vi "Picture_View_ROI.vi"(8 "Input Cluster":T6, 10 "ROI":bool, 11 "Cluster 2":T7) -> (0 "ROI-Picture":i32[][](array[numeric]), 3 "Out of range":bool[](array[boolean]))   [LabVIEW 2009]
uses:
  atmcd32d.llb/AcquisitionMode_mode typedef.ctl
  atmcd32d.llb/ReadMode_mode typedef.ctl
  atmcd32d.llb/TriggerMode_mode typedef.ctl
  atmcd32d.llb/Shutter_type typedef.ctl
  atmcd32d.llb/Shutter_mode typedef.ctl
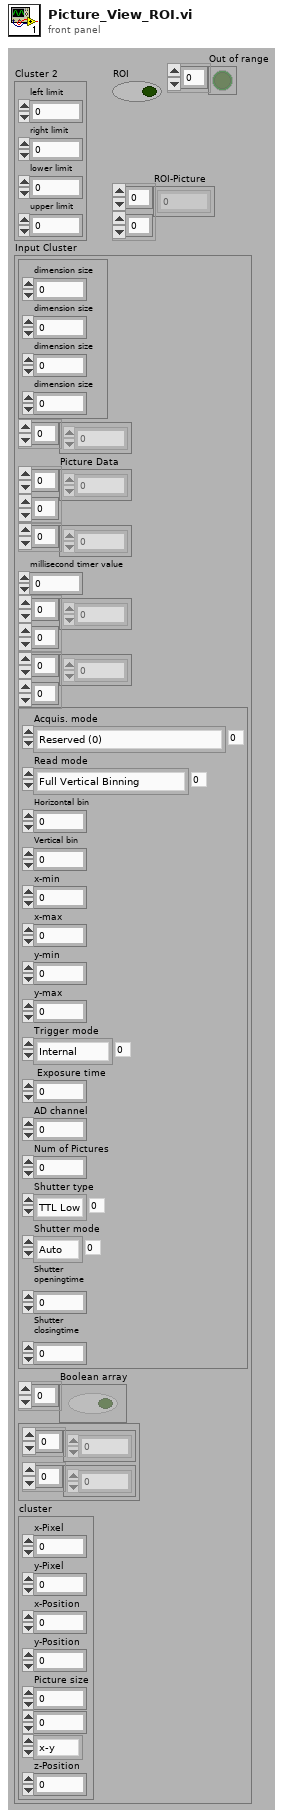
[diagram p1: front panel]
types:
  T1 = typedef "AcquisitionMode_mode typedef.ctl" = enum16{"Reserved (0)", "Single Scan", "Accumulate", "Kinetics", "Fast Kinetics", "Run Till Abort", "Reserved (6)", "Reserved (7)", "Reserved (8)", "Time Delayed Integration"}
  T2 = typedef "ReadMode_mode typedef.ctl" = enum16{"Full Vertical Binning", "Multi-Track", "Random-Track", "Single-Track", "Image"}
  T3 = typedef "TriggerMode_mode typedef.ctl" = enum16{"Internal", "External", "N/A (2)", "N/A (3)", "N/A (4)", "N/A (5)", "External Start"}
  T4 = typedef "Shutter_type typedef.ctl" = enum16{"TTL Low", "TTL High"}
  T5 = typedef "Shutter_mode typedef.ctl" = enum16{"Auto", "Open", "Close"}
  T6 = cluster{cluster{"dimension size":i32, "dimension size":i32, "dimension size":i32, "dimension size":i32}, i32[], "Picture Data":dbl[][], u32[], "millisecond timer value":u32, dbl[][], i32[][], cluster{"Acquis. mode":T1, "Read mode":T2, "Horizontal bin":i32, "Vertical bin":i32, "x-min":i32, "x-max":i32, "y-min":i32, "y-max":i32, "Trigger mode":T3, " Exposure time":sgl, "AD channel":i32, "Num of Pictures":i32, "Shutter type":T4, "Shutter mode":T5, "Shutter\nopeningtime":i32, "Shutter\nclosingtime":i32}, "Boolean array":bool[], cluster{dbl[], dbl[]}, "cluster":cluster{"x-Pixel":u16, "y-Pixel":u16, "x-Position":dbl, "y-Position":dbl, "Picture size":dbl, dbl, enum32{"x-y", "x-z", "y-z"}, "z-Position":dbl}}
  T7 = cluster{"left limit":i32, "right limit":i32, "lower limit":i32, "upper limit":i32}
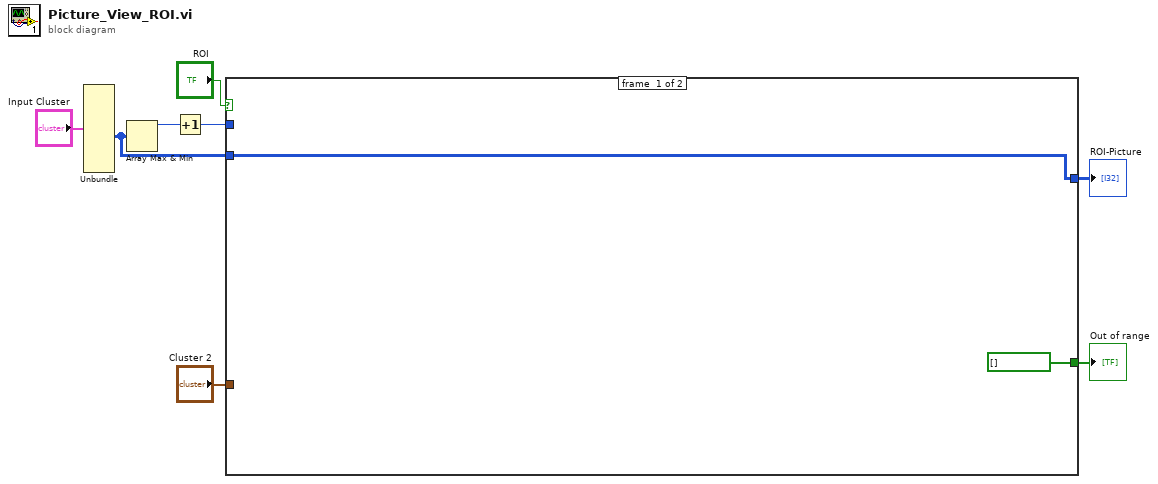
[diagram p0: block diagram]
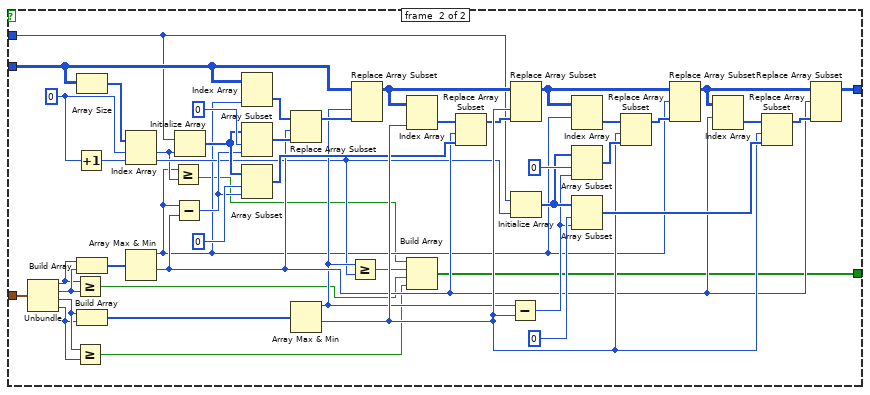
[diagram p2: hidden frame]
diagram:
  n1 = Unbundle("Input Cluster") -> (w4:i32[][])  [unwired: 10 out]
  n2 = Array Max & Min(array=w4) -> (max value=w6:i32)  [unwired: 3 out]
  n3 = Increment(x=w6) -> (x+1=w5:i32)
  n4 = case shown="True" "ROI" {
    tunnel: w4 -> [w10 w32]
    tunnel: [w10 w52] -> w3
    tunnel: "Cluster 2" -> [_ w25]
    tunnel: w5 -> [_ w24]
    tunnel: [bool[] [] w11] -> w1
    frame #0 {
    }
    frame #1 {
      w54 = 0 ("index")
      n5 = Unbundle(w25) -> ("left limit"=w17:i32, "right limit"=w20:i32, "lower limit"=w19:i32, "upper limit"=w18:i32)
      n6 = Greater Or Equal?(x=w17, y=w20) -> (x >= y?=w14:bool)
      n7 = Greater Or Equal?(x=w19, y=w18) -> (x >= y?=w15:bool)
      n8 = Increment(x=w54) -> (x+1=w55:i32)
      n9 = Array Size(array=w32) -> (size(s)=w56:i32[])
      n10 = Build Array(w17, w20) -> (w53:i32[])
      n11 = Build Array(w19, w18) -> (w57:i32[])
      n12 = Index Array(array=w56, index #1=w54, index #2=w55) -> (element #1=w21:i32, element #2=w22:i32)
      n13 = Array Max & Min(array=w53) -> (max value=w16:i32, min value=w26:i32)  [unwired: 2 out]
      n14 = Greater Or Equal?(x=w16, y=w21) -> (x >= y?=w12:bool)
      n15 = Subtract(x=w16, y=w26) -> (x-y=w27:i32)
      n16 = Initialize Array(w24, w21) -> (w28:i32[])
      n17 = Index Array(array=w32, index (col)=w16) -> (element=w31:i32[])  [unwired: 1 in]
      n18 = Array Subset(array=w28, index=0, length=w27) -> (w29:i32[])
      n19 = Array Subset(array=w28, index=0, length=w27) -> (w34:i32[])
      n20 = Replace Array Subset(array=w31, new element=w29, index=w26) -> (w33:i32[])
      n21 = Array Max & Min(array=w57) -> (max value=w23:i32, min value=w38:i32)  [unwired: 2 out]
      n22 = Greater Or Equal?(x=w23, y=w22) -> (x >= y?=w13:bool)
      n23 = Replace Array Subset(array=w32, new element=w33, index (col)=w23) -> (w39:i32[][])  [unwired: 1 in]
      n24 = Index Array(array=w39, index (col)=w38) -> (element=w36:i32[])  [unwired: 1 in]
      n25 = Build Array(w12, w13, w14, w15) -> (w11:bool[])
      n26 = Replace Array Subset(array=w36, new element=w34, index=w26) -> (w35:i32[])
      n27 = Subtract(x=w23, y=w38) -> (x-y=w41:i32)
      n28 = Replace Array Subset(array=w39, new element=w35, index (col)=w38) -> (w46:i32[][])  [unwired: 1 in]
      n29 = Initialize Array(w24, w22) -> (w43:i32[])
      n30 = Index Array(array=w46, index (row)=w16) -> (element=w45:i32[])  [unwired: 1 in]
      n31 = Array Subset(array=w43, index=0, length=w41) -> (w42:i32[])
      n32 = Array Subset(array=w43, index=0, length=w41) -> (w48:i32[])
      n33 = Replace Array Subset(array=w45, new element=w42, index=w38) -> (w40:i32[])
      n34 = Replace Array Subset(array=w46, new element=w40, index (row)=w16) -> (w51:i32[][])  [unwired: 1 in]
      n35 = Index Array(array=w51, index (row)=w26) -> (element=w50:i32[])  [unwired: 1 in]
      n36 = Replace Array Subset(array=w50, new element=w48, index=w38) -> (w47:i32[])
      n37 = Replace Array Subset(array=w51, new element=w47, index (row)=w26) -> (w52:i32[][])  [unwired: 1 in]
    }
  }
  "ROI-Picture" <- w3
  "Out of range" <- w1
